vi "FPGA Main_config-V2.vi"() -> ()   [LabVIEW 2015]
doc: "This FPGA Main VI contains a control loop running in parallel with an RT watchdog loop.\n- The Control Loop performs control calculations on four input channels in parallel, and outputs the results to four output channels.\n- The RT Watchdog Loop checks for a periodic 'pet' from the RT Main VI to ensure communications between RT and FPGA are maintained."
uses:
  <vilib>/LabVIEW Targets/FPGA/cRIO/shared/nicrio_ModuleControls/nicrio_cRIO-9234_DataRatesRing2.ctl
  <vilib>/LabVIEW Targets/FPGA/cRIO/shared/nicrio_ModuleControls/nicrio_cRIO-9234_ConfigModeRing.ctl
  <vilib>/rvi/Emulation/niFpgaGetClockAttributes.vi
  <vilib>/rvi/Emulation/niFpgaSctlEmulationGetInTimedLoop.vi
  <vilib>/rvi/Emulation/niFpgaEmulationReportErrorSimple.vi
  <vilib>/rvi/Emulation/niFpgaProcessEmulError.vi
  <vilib>/rvi/eio/common/nirviEmuTemplatePropertySet_errors.vi
  <vilib>/rvi/eio/common/nirviEmuTemplateMethod_errors.vi
  <vilib>/rvi/interface/RandomDataEmulation/niFpgaRandomDataHandleErrors.vi
  <vilib>/rvi/Emulation/niFpgaCriticalErrorInLSC.vi
  <vilib>/eio/EIOPropertyNode/EIOPropertyNode.xnode
  <vilib>/eio/EIONode/EIONode.xnode
  <vilib>/rvi/DataTransferAndStorage/Container/XNode/niFpgaContainer.xnode
  <vilib>/rvi/interface/RandomDataEmulation/nirviRandomDataFpgaReadWriteTemplate.vi
  <vilib>/rvi/eio/common/nirviEmuTemplatePropertyGet_errors.vi
  <vilib>/rvi/eio/common/nirviEmuTemplatePropertyGet_noerrors.vi
  <vilib>/rvi/eio/common/nirviEmuTemplatePropertySet_noerrors.vi
panel:
  in  "Input Configuration Array":T1[](array[typedef])=[0, 0, 0, 0] items=["AC Coupled", "DC Coupled", "IEPE AC Coupled"]
  in  "Data Rate":T2=1 items=["51.200 kS/s (NI 9234)"=1, "25.600 kS/s (NI 9234)"=2, "17.067 kS/s (NI 9234)"=3, "12.800 kS/s (NI 9234)"=4, "10.240 kS/s (NI 9234)"=5, "8.533 kS/s (NI 9234)"=6, "7.314 kS/s (NI 9234)"=7, "6.400 kS/s (NI 9234)"=8, "5.689 kS/s (NI 9234)"=9, "5.120 kS/s (NI 9234)"=10, "4.654 kS/s (NI 9234)"=11, "4.267 kS/s (NI 9234)"=12, "3.938 kS/s (NI 9234)"=13, "3.657 kS/s (NI 9234)"=14, "3.413 kS/s (NI 9234)"=15, "3.200 kS/s (NI 9234)"=16, "3.012 kS/s (NI 9234)"=17, "2.845 kS/s (NI 9234)"=18, "2.695 kS/s (NI 9234)"=19, "2.560 kS/s (NI 9234)"=20, "2.438 kS/s (NI 9234)"=21, "2.328 kS/s (NI 9234)"=22, "2.226 kS/s (NI 9234)"=23, "2.133 kS/s (NI 9234)"=24, "2.048 kS/s (NI 9234)"=25, "1.969 kS/s (NI 9234)"=26, "1.896 kS/s (NI 9234)"=27, "1.829 kS/s (NI 9234)"=28, "1.765 kS/s (NI 9234)"=29, "1.707 kS/s (NI 9234)"=30, "1.652 kS/s (NI 9234)"=31]
  out "FPGA Error":errorcluster
  out "Finished":bool
  in  "Stop":bool
  out "Module Underflow":bool
  out "DMA FIFO Full":bool
  out "Different Channel Count":bool
  out "Actual Loop Period (ticks)":u32
  out "First Read":bool
  in  "Number of Channels":i32=4
  in  "Channel Scale Array":fxp<+,24,12>[](array[numeric])=[0.0, 0.0, 0.0, 0.0]
  # "General Settings"
  # "Monitoring Values"
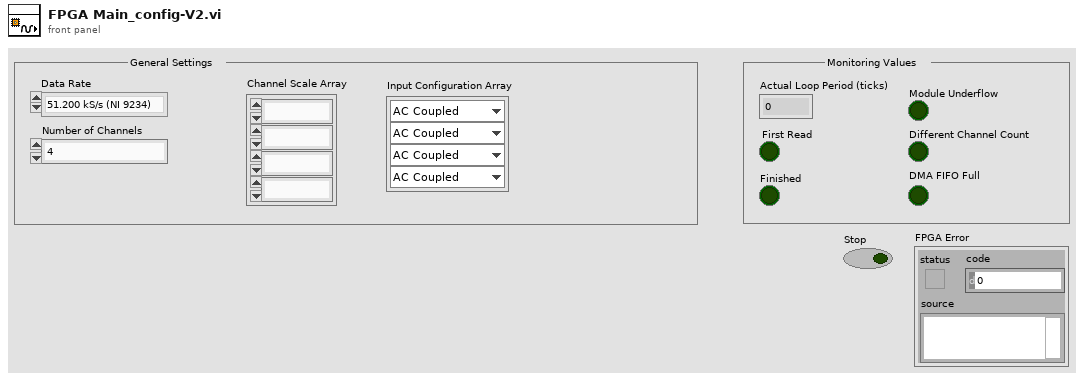
[diagram p1: front panel]
types:
  T1 = typedef "nicrio_cRIO-9234_ConfigModeRing.ctl" = u8
  T2 = typedef "nicrio_cRIO-9234_DataRatesRing2.ctl" = u8
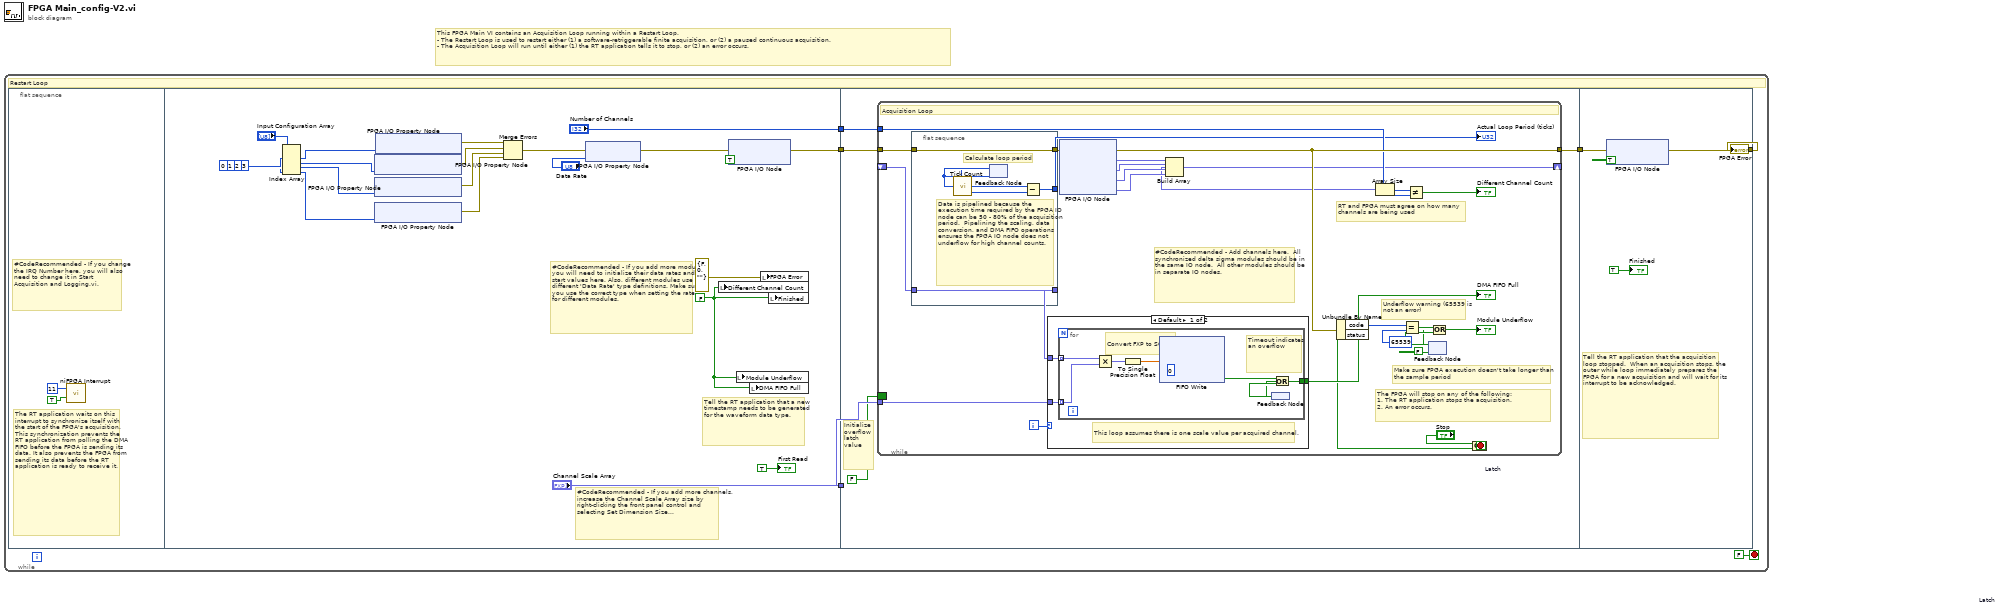
[diagram p0: block diagram]
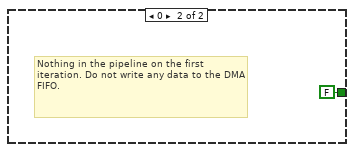
[diagram p2: hidden frame]
diagram:
  # "This FPGA Main VI contains an Acquisition Loop running within a Restart Loop.\n- The Restart Loop is used to restart either (1) a software-retriggerable finite acquisition, or (2) a paused continuous acquisition.\n- The Acquisition Loop will run until either (1) the RT application tells it to stop, or (2) an error occurs."
  n1 = while {
    stop <- FALSE stop-if-true
    # "Restart Loop"
    n2 = flat-sequence {
      tunnel: [w31] -> w5
      tunnel: ["Channel Scale Array"] -> w4
      tunnel: ["Number of Channels"] -> w3
      tunnel: w5 -> [w35]
      tunnel: w4 -> [w34]
      tunnel: w3 -> [w36]
      tunnel: [w33] -> w2
      tunnel: w2 -> [w81]
      tunnel: [w80] -> w1
      frame #0 {
        # "#CodeRecommended - If you change the IRQ Number here, you will also need to change it in Start Acquisition and Logging.vi."
        # "The RT application waits on this interrupt to synchronize itself with the start of the FPGA's acquisition.  This synchronization prevents the RT application from polling the DMA FIFO before the FPGA is sending its data. It also prevents the FPGA from sending its data before the RT application is ready to receive it."
        n3 = call <vilib>:"niFPGA Interrupt.vi"("Wait Until Cleared (F)"=TRUE ("Wait Until Cleared"), "IRQ Number (0)"=u8 11 ("IRQ Number")) -> ()  [unwired: 1 in]
      }
      frame #1 {
        w28 = FALSE ("Module Underflow")
        # "Tell the RT application that a new timestamp needs to be generated for the waveform data type."
        # "#CodeRecommended - If you add more channels, increase the Channel Scale Array size by right-clicking the front panel control and selecting Set Dimension Size..."
        # "#CodeRecommended - If you add more modules, you will need to initialize their data rates and start values here. Also, different modules use different 'Data Rate' type definitions. Make sure you use the correct type when setting the rate for different modules."
        n4 = Index Array(array="Input Configuration Array", index #1=0 ("index"), index #2=1 ("index"), index #3=2 ("index"), index #4=3 ("index")) -> (element #1=w15:T1, element #2=w14:T1, element #3=w13:T1, element #4=w12:T1)
        n5 = xnode "FPGA I/O Property Node"("Input Configuration"=w14) -> ("error out"=w21:errorcluster)  [unwired: 2 in, 1 out]
        n6 = xnode "FPGA I/O Property Node"("Input Configuration"=w13) -> ("error out"=w20:errorcluster)  [unwired: 2 in, 1 out]
        n7 = xnode "FPGA I/O Property Node"("Input Configuration"=w12) -> ("error out"=w19:errorcluster)  [unwired: 2 in, 1 out]
        n8 = xnode "FPGA I/O Property Node"("Input Configuration"=w15) -> ("error out"=w22:errorcluster)  [unwired: 2 in, 1 out]
        n9 = Merge Errors(w22, w21, w20, w19) -> (w18:errorcluster)
        n10 = xnode "FPGA I/O Property Node"("error in"=w18, "Data Rate"="Data Rate") -> ("error out"=w23:errorcluster)  [unwired: 1 in, 1 out]
        n11 = local write "Different Channel Count"(w28) -> ()
        n12 = xnode "FPGA I/O Node"("error in"=w23, "Mod1/Start"=TRUE) -> ("error out"=w31:errorcluster)  [unwired: 1 in, 1 out]
        n13 = local write "Module Underflow"(w28) -> ()
        n14 = local write "DMA FIFO Full"(w28) -> ()
        n15 = local write "FPGA Error"(errorcluster {"status"=FALSE, "code"=0, "source"=""} ("FPGA Error")) -> ()
        n16 = local write "Finished"(w28) -> ()
        "First Read" <- TRUE ("First Read")
      }
      frame #2 {
        # "Initialize overflow latch value"
        n17 = while {
          tunnel: w35 -> [w54]
          tunnel: [w59] -> w33
          shift-right: [w44] -> _
          shift-left: _ -> [w46]
          tunnel: w36 -> [w56]
          tunnel: w34 -> [w48]
          border: FALSE ("Overflow\nLatch") -> [_]
          i -> [w37]
          stop <- w62 stop-if-true
          # "Underflow warning (65539 is not an error)"
          # "The FPGA will stop on any of the following:\n1. The RT application stops the acquisition.\n2. An error occurs."
          # "#CodeRecommended - Add channels here.  All synchronized delta sigma modules should be in the same IO node.  All other modules should be in separate IO nodes."
          # "RT and FPGA must agree on how many channels are being used"
          # "Make sure FPGA execution doesn't take longer than the sample period"
          # "Acquisition Loop"
          n18 = flat-sequence {
            tunnel: [w79] -> w53
            tunnel: w54 -> [w79]
            tunnel: [w76] -> w52
            tunnel: w46 -> [w75]
            tunnel: [w75] -> w47
            frame #0 {
              # "Data is pipelined because the execution time required by the FPGA IO node can be 50 - 80% of the acquisition period.  Pipelining the scaling, data conversion, and DMA FIFO operations ensures the FPGA IO node does not underflow for high channel counts."
              # "Calculate loop period"
              n19 = call "Tick Count"() -> ("Tick Count(Ticks)"=w78:u32)
              n20 = feedback-in #1(w78) -> ()
              n21 = feedback #1(w78) -> (w77:u32)
              n22 = Subtract(x=w78, y=w77) -> (x-y=w76:u32)
            }
          }
          n23 = case shown="Default" w37 {
            tunnel: [w65 FALSE] -> w58
            tunnel: w48 -> [w64 _]
            tunnel: w47 -> [w63 _]
            frame Default {
              # "This loop assumes there is one scale value per acquired channel."
              n24 = for {
                tunnel: [w71] -> w65
                tunnel: w63 -> [w69] mode=indexing
                tunnel: w64 -> [w68] mode=indexing
                # "Timeout indicates an overflow"
                # "Convert FXP to SGL"
                n25 = Multiply(x=w69, y=w68) -> (x*y=w67:fxp<+/-,48,16>)
                n26 = To Single Precision Float(number=w67) -> (single precision float=w66:sgl)
                n27 = xnode ("FIFO Write")("Element"=w66, "Timeout"=0) -> ("Timed Out?"=w73:bool)  [unwired: 1 in, 1 out]
                n28 = feedback #2 "Latch"() -> (w72:bool)
                n29 = Or(x=w73, y=w72) -> (x .or. y?=w71:bool)
                n30 = feedback-in #2(w71) -> ()
              }
            }
            frame 0 {
              # "Nothing in the pipeline on the first iteration. Do not write any data to the DMA FIFO."
            }
          }
          "DMA FIFO Full" <- w58
          n31 = xnode "FPGA I/O Node"("error in"=w53) -> ("error out"=w59:errorcluster, "Mod1/AI0"=w51:fxp<+/-,24,4>, "Mod1/AI1"=w45:fxp<+/-,24,4>, "Mod1/AI2"=w50:fxp<+/-,24,4>, "Mod1/AI3"=w49:fxp<+/-,24,4>)  [unwired: 4 in, 4 out]
          n32 = Build Array(w51, w45, w50, w49) -> (w44:fxp<+/-,24,4>[])
          n33 = Unbundle By Name(w59) -> ("code"=w60:i32, "status"=w39:bool)
          n34 = Array Size(array=w44) -> (size(s)=w57:i32)
          n35 = Equal?(x=w60, y=65539) -> (x = y?=w41:bool)
          n36 = Not Equal?(x=w57, y=w56) -> (x != y?=→"Different Channel Count":bool)
          n37 = feedback #3 "Latch"(FALSE) -> (w43:bool)
          n38 = Or(x=w41, y=w43) -> (x .or. y?=w40:bool)
          "Module Underflow" <- w40
          n39 = feedback-in #3(w40) -> ()
          n40 = Compound Arithmetic op=OR("Stop", w39) -> (w62:bool)
          "Actual Loop Period (ticks)" <- w52
        }
      }
      frame #3 {
        # "Tell the RT application that the acquisition loop stopped.  When an acquisition stops, the outer while loop immediately prepares the FPGA for a new acquisition and will wait for its interrupt to be acknowledged."
        n41 = xnode "FPGA I/O Node"("error in"=w81, "Mod1/Stop"=TRUE) -> ("error out"=w80:errorcluster)  [unwired: 1 in, 1 out]
        "Finished" <- TRUE ("Finished")
      }
    }
    "FPGA Error" <- w1
  }
